vi "ParseSWI.vi"(8 "error in (no error)":errorcluster, 9 "Master Device in":refnum<class "Master Device.lvclass">, 10 "Current Variables":T1[](array[typedef]), 11 "Arduino in":refnum<class "Arduino.lvclass">) -> (0 "error out":errorcluster, 2 "Master Device out":refnum<class "Master Device.lvclass">, 3 "Arduino out":refnum<class "Arduino.lvclass">)   [LabVIEW 2013, in "Arduino.lvclass"]
doc: "All specific devices will override ParseSWI method (i.e. you can delete the parent call)\n (1) Get devices data from private data\n (2) Get Slave Info (Ramp List) from Master Device\n (3) Parse data into \"prepared HWI\" which is in reverse order to match Ramp List."
uses:
  Arduino.lvclass
  Master Device/Master Device.lvclass
  TypeDefs/Active procedure variables.ctl
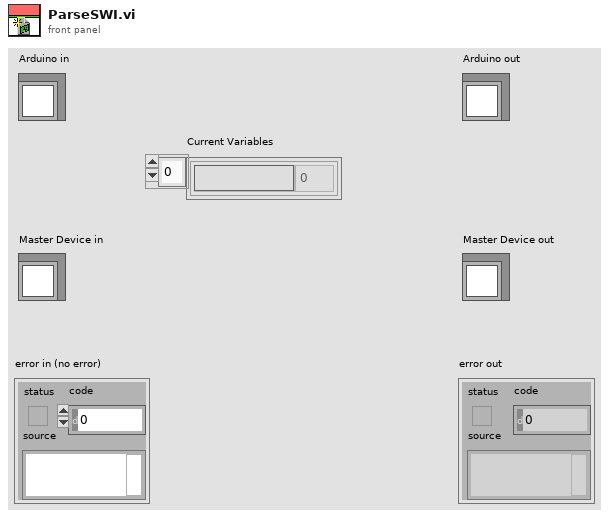
[diagram p1: front panel]
types:
  T1 = typedef "Active procedure variables.ctl" = cluster{"Procedure variable":string, "Value":dbl}
  T2 = cluster{"Array":cluster{"Short Command":string, "ParamTotal":dbl, "Params":dbl[]}[]}
  T3 = cluster{"Short Command":string, "ParamTotal":dbl, "Params":dbl[]}
  T4 = cluster{"Name":string, "Allowed Functions":cluster{"Display Name":string, "Short Command":string, "Number of Args":dbl}[]}[]
  T5 = cluster{"Display Name":string, "Short Command":string, "Number of Args":dbl}[]
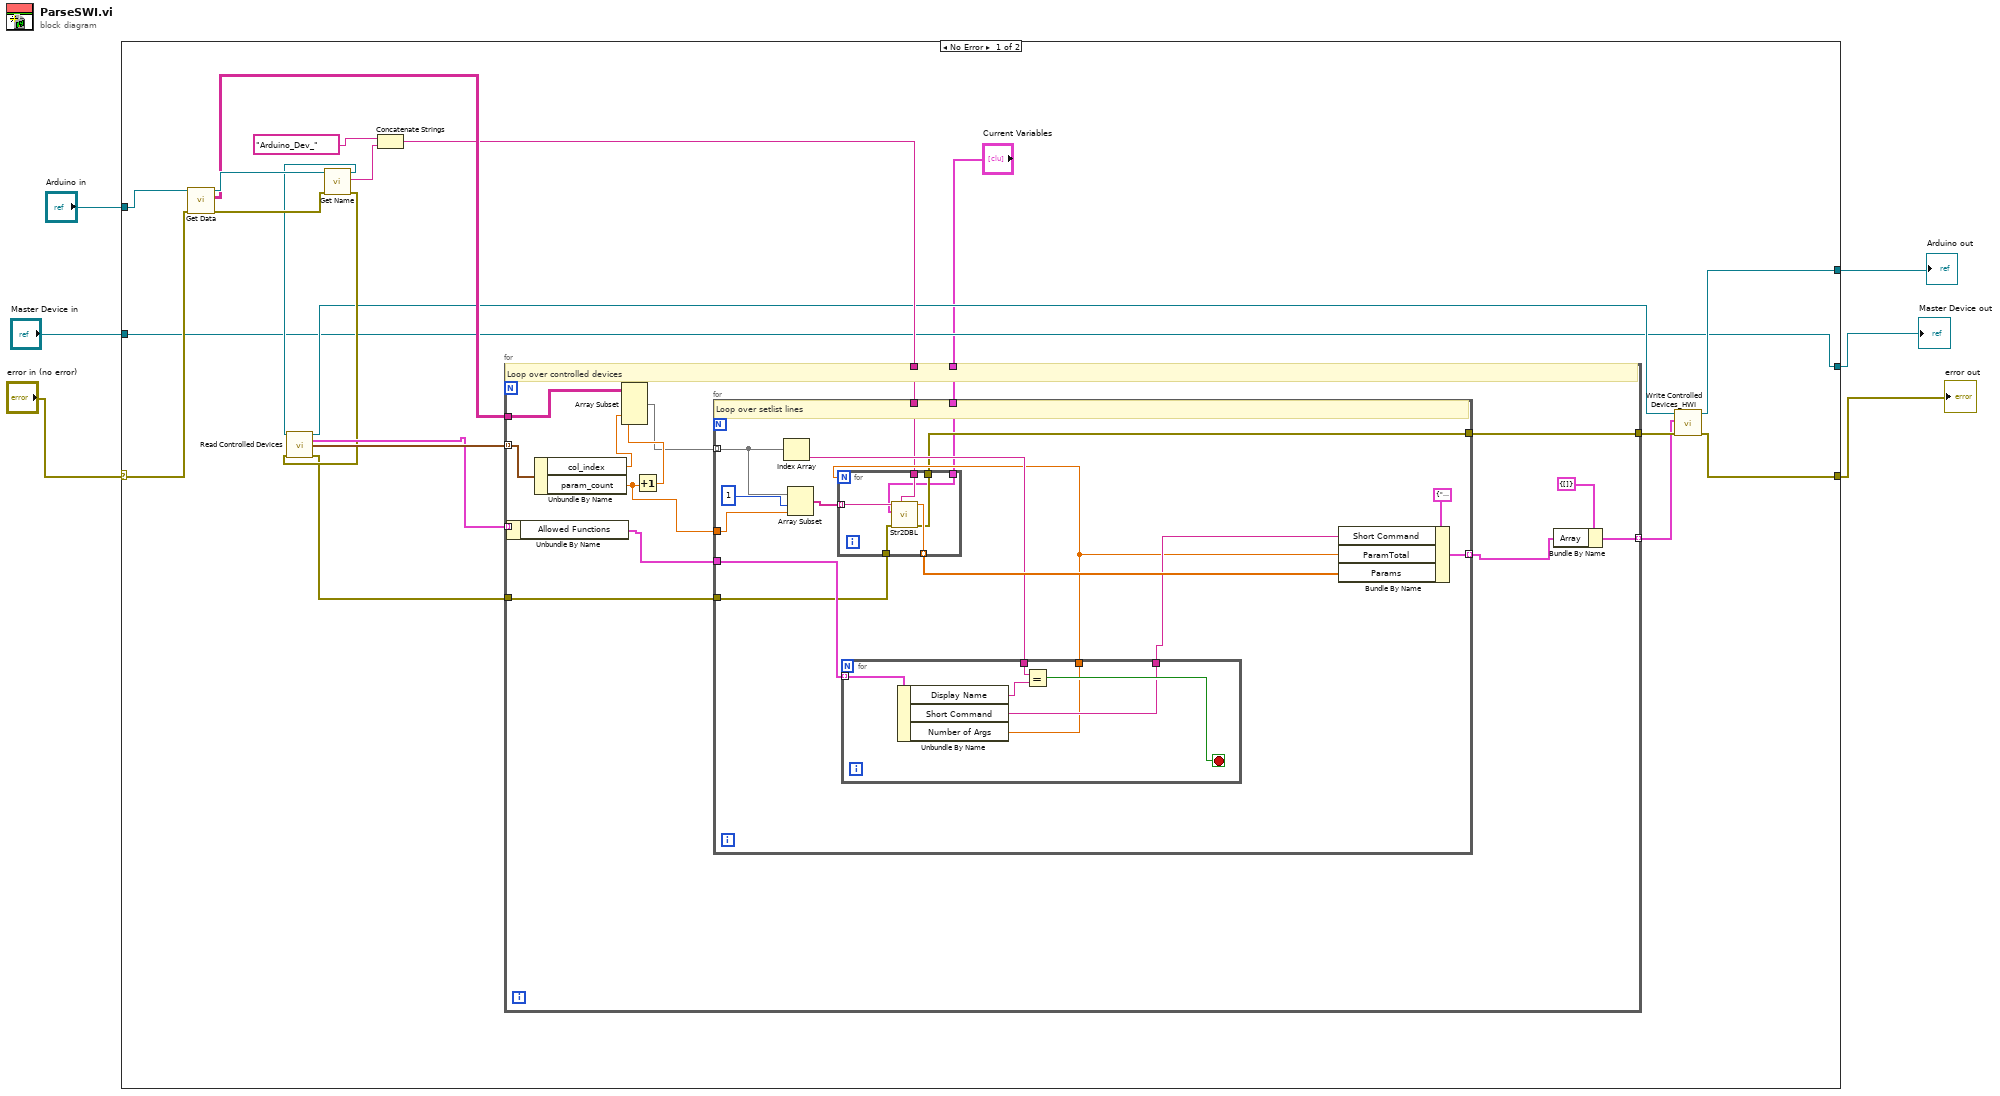
[diagram p0: block diagram]
diagram:
  n1 = case shown="No Error" "error in (no error)" {
    selector: "error in (no error)" -> [w22 w71]
    tunnel: [w10 w71] -> w5
    tunnel: [w9 w70] -> w4
    tunnel: "Master Device in" -> [w9 w70]
    tunnel: [w11 w69] -> w2
    tunnel: "Arduino in" -> [w24 w69]
    frame No Error {
      n2 = call-dynamic "Get Data.vi"("error in (no error)"=w22, "Device in"=w24) -> ("error out"=w21:errorcluster, "Table Indicator"=w19:string[][], "Device out"=w23:refnum<class "Arduino.lvclass">)  [unwired: 6 in]
      n3 = call-dynamic "Get Name.vi"("error in (no error)"=w21, "Device in"=w23) -> ("error out"=w15:errorcluster, "Name"=w25:string, "Device out"=w20:refnum<class "Arduino.lvclass">)  [unwired: 7 in]
      n4 = call-dynamic "Read Controlled Devices.vi"("Arduino in"=w20, "error in (no error)"=w15) -> ("Arduino out"=w12:refnum<class "Arduino.lvclass">, "Controlled Devices"=w17:T4, "Device Cols"=w18:cluster{"col_index":dbl, "param_count":dbl}[], "error out"=w14:errorcluster)  [unwired: 10 in]
      n5 = Concatenate Strings("Arduino_Dev_", w25) -> (w16:string)
      n6 = for {
        tunnel: w19 -> [w41]
        tunnel: w18 -> [w40] mode=indexing
        tunnel: w17 -> [w35] mode=indexing
        tunnel: [w31] -> w7 mode=indexing
        tunnel: w16 -> [w30]
        tunnel: w14 -> [w29]
        tunnel: [w28] -> w13
        tunnel: "Current Variables" -> [w27]
        # "Loop over controlled devices"
        n7 = Unbundle By Name(w35) -> ("Allowed Functions"=w34:T5)
        n8 = Unbundle By Name(w40) -> ("col_index"=w39:dbl, "param_count"=w36:dbl)
        n9 = Increment(x=w36) -> (x+1=w38:dbl)
        n10 = Array Subset(array=w41, index (col)=w39, length (col)=w38) -> (w37:string[][])  [unwired: 2 in]
        n11 = for {
          tunnel: w37 -> [w56] mode=indexing
          tunnel: w36 -> [w55]
          tunnel: w34 -> [w51]
          tunnel: [w47] -> w32 mode=indexing
          tunnel: w30 -> [w46]
          tunnel: w29 -> [w45]
          tunnel: [w44] -> w28
          tunnel: w27 -> [w43]
          # "Loop over setlist lines"
          n12 = Index Array(array=w56) -> (element=w50:string)  [unwired: 1 in]
          n13 = Array Subset(array=w56, index=1, length=w55) -> (w54:string[])
          n14 = for {
            tunnel: w51 -> [w62] mode=indexing
            tunnel: [w59] -> w49
            tunnel: [w58] -> w48
            tunnel: w50 -> [w57]
            stop <- w60 stop-if-true
            n15 = Unbundle By Name(w62) -> ("Display Name"=w61:string, "Short Command"=w59:string, "Number of Args"=w58:dbl)
            n16 = Equal?(x=w57, y=w61) -> (x = y?=w60:bool)
          }
          n17 = for {
            N: w48 -> [_]
            tunnel: w54 -> [w68] mode=indexing
            tunnel: [w67] -> w52 mode=indexing
            tunnel: w46 -> [w66]
            tunnel: w45 -> [w65]
            tunnel: [w64] -> w44
            tunnel: w43 -> [w63]
            n18 = call "Str2DBL.vi"("Error Locator"=w66, "error in (no error)"=w65, "Current Variable settings"=w63, "formula"=w68) -> ("error out"=w64:errorcluster, "y value"=w67:dbl)  [unwired: 4 in]
          }
          n19 = Bundle By Name(cluster=T3 {"Short Command"="", "ParamTotal"=0.0, "Params"=[]} ("Line"), "Short Command"=w49, "ParamTotal"=w48, "Params"=w52) -> (w47:T3)
        }
        n20 = Bundle By Name(cluster=T2 {"Array"=[]} ("Device SetList"), "Array"=w32) -> (w31:T2)
      }
      n21 = call-dynamic "Write Controlled Devices_HWI.vi"("error in (no error)"=w13, "Controlled Devices"=w7, "Arduino in"=w12) -> ("error out"=w10:errorcluster, "Arduino out"=w11:refnum<class "Arduino.lvclass">)  [unwired: 7 in]
    }
    frame Error {
    }
  }
  "error out" <- w5
  "Arduino out" <- w2
  "Master Device out" <- w4
